vi "waveform_to_tdms.vi"(4 "waveform":waveform(dbl)) -> (1 "appended time data":dbl[][](array[numeric]))   [LabVIEW 2011]
doc: "calculates the timing info for a waveform an ouputs a 2D array consisting of the time and the amplitude info."
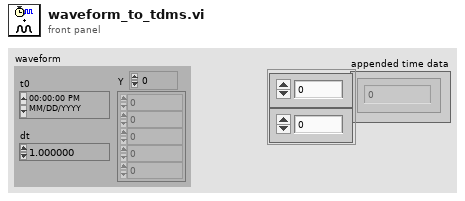
[diagram p1: front panel]
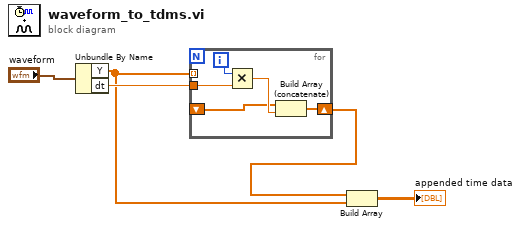
[diagram p0: block diagram]
diagram:
  n1 = Unbundle By Name("waveform") -> ("Y"=w3:dbl[], "dt"=w5:dbl)
  n2 = for {
    tunnel: w5 -> [w7]
    shift-right: [w10] -> w4
    shift-left: _ -> [w8]
    tunnel: w3 -> [_] mode=indexing
    i -> [w6]
    n3 = Multiply(x=w6, y=w7) -> (x*y=w9:dbl)
    n4 = Build Array (concatenate)(w8, w9) -> (w10:dbl[])
  }
  n5 = Build Array(w4, w3) -> (→"appended time data":dbl[][])
